vi "ReadDriveEncoder.vi"() -> ()   [LabVIEW 2013]
uses:
  RefnameEnum.ctl
  Sally_Dashboard_2014/DBNameEnum.ctl
  Robot Global Data.vi
panel:
  out "DistanceR (in)":dbl
  out "EncoderR Rate (deg/sec)":dbl
  in  "Reset EncoderR?":bool
  in  "Reset EncoderL?":bool
  out "EncoderL Rate (deg/sec)":dbl
  out "DistanceL (in)":dbl
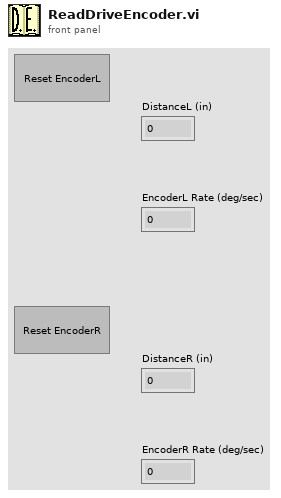
[diagram p1: front panel]
types:
  T1 = typedef "RefnameEnum.ctl" = enum16{"FireLauncher", "Climber", "Shield", "TankDrive", "DriveEncoderL", "DriveEncoderR", "LauncherMotorRPM", "LauncherEncoderAnalog", "LauncherEncoderRPM", "ShooterLS", "DriveAlignLSLeft", "DriveAlignLSRight", "ClimbingLS", "LauncherEncoderAngle", "LauncherMotorAngle", "Gamepad1", "Gamepad2", "Compressor", "ClimbWeightSol3", "ClimbWeightSol4"}
  T2 = typedef "WPI_EncoderDevRef.ctl" = cluster{"DevStatus":errorcluster, "EncoderIndex":T3, "CounterIndex":T4, "DistancePerCount":dbl, "Decoding Type":T5}
  T3 = typedef "FPGA_EncoderIdx.ctl" = enum8{"Enc 0", "Enc 1", "Enc 2", "Enc 3", "Invalid"}
  T4 = typedef "FPGA_CounterCtrSystemIndex.ctl" = enum8{"Ctr 0", "Ctr 1", "Ctr 2", "Ctr 3", "Ctr 4", "Ctr 5", "Ctr 6", "Ctr 7", "Invalid"}
  T5 = typedef "WPI_EncoderType.ctl" = enum16{"1x", "2x", "4x"}
  T6 = typedef "DBNameEnum.ctl" = enum16{"AutoInstructions", "DriveLoopTime", "DriveAlignLSLeft", "DriveAlignLSRight", "Use2DriveAlign", "ClimbLS", "LauncherAngleMatches", "FrameworkVersion", "sLauncherAngle", "LauncherTargetAngle", "sLauncherRPM", "LauncherTargetRPM", "sDriveDistance", "LauncherMotorValue", "PullbackTol", "FireTol", "LauncherRPMTol", "LauncherAngleTol", "InitialWait", "WaitBetweenLaunch", "AnglePresets", "RPMPresets", "UseAngleEncoder", "UseLauncherEncoder", "UseLauncherPID", "QSWaitBeforeFire", "QSWaitBeforeRetract", "AngleForwardValue", "AngleBackwardValue", "UseClusterArray", "BackupAuto", "ReverseDriveIndicate", "HalfSpeedFactor"}
  T7 = typedef "LoopDisable.ctl" = cluster{"Climb.vi":bool, "LauncherAngle.vi":bool, "Launcher.vi":bool, "ArmControl.vi":bool, "WinchMotor.vi":bool, "ReadDriveEncoder.vi":bool}
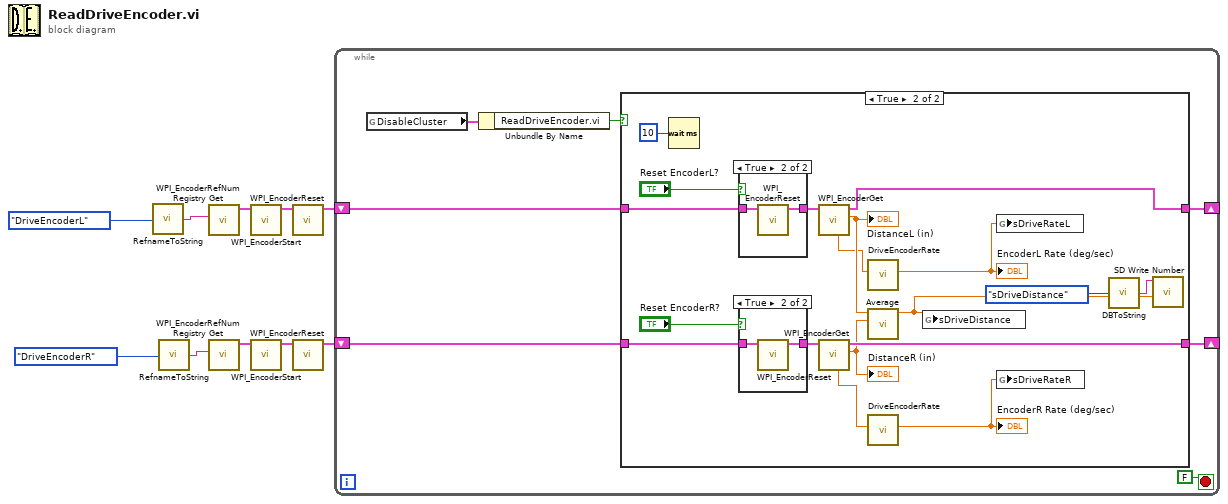
[diagram p0: block diagram]
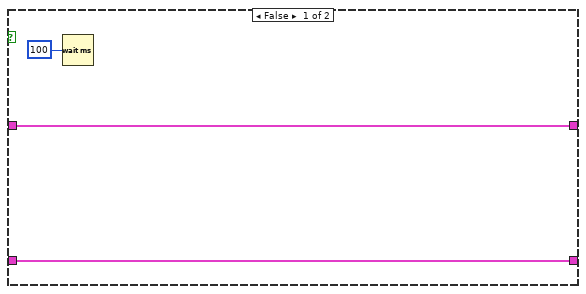
[diagram p2: hidden frame]
diagram:
  n1 = call "RefnameToString.vi"("Enum"=RefnameEnum."DriveEncoderL") -> ("Refname"=w2:string)
  n2 = call "RefnameToString.vi"("Enum"=RefnameEnum."DriveEncoderR") -> ("Refname"=w1:string)
  n3 = call <vilib>:"WPI_EncoderRefNum Registry Get.vi"("refnum name"=w2) -> ("EncoderDevRef"=w10:T2)  [unwired: 9 in, 1 out]
  n4 = call <vilib>:"WPI_EncoderRefNum Registry Get.vi"("refnum name"=w1) -> ("EncoderDevRef"=w7:T2)  [unwired: 9 in, 1 out]
  n5 = call <vilib>:"WPI_EncoderStart.vi"("EncoderDevRef"=w10) -> ("EncoderDevRef"=w9:T2)  [unwired: 1 in, 9 out]
  n6 = call <vilib>:"WPI_EncoderStart.vi"("EncoderDevRef"=w7) -> ("EncoderDevRef"=w6:T2)  [unwired: 1 in, 9 out]
  n7 = call <vilib>:"WPI_EncoderReset.vi"("EncoderDevRef"=w9) -> ("EncoderDevRef"=w8:T2)  [unwired: 1 in, 9 out]
  n8 = call <vilib>:"WPI_EncoderReset.vi"("EncoderDevRef"=w6) -> ("EncoderDevRef"=w5:T2)  [unwired: 1 in, 9 out]
  n9 = while {
    shift-right: [w15] -> _
    shift-left: w8 -> [w16]
    shift-right: [w14] -> _
    shift-left: w5 -> [w13]
    stop <- FALSE stop-if-true
    n10 = global read "Robot Global Data.vi" "DisableCluster"() -> (w12:T7)
    n11 = Unbundle By Name(w12) -> ("ReadDriveEncoder.vi"=w11:bool)
    n12 = case shown="True" w11 {
      tunnel: w16 -> [w20 w37]
      tunnel: [w20 w35] -> w15
      tunnel: [w19 w33] -> w14
      tunnel: w13 -> [w19 w32]
      frame False {
        n13 = Wait (ms)(milliseconds to wait=u32 100) -> ()  [unwired: 1 out]
      }
      frame True {
        n14 = Wait (ms)(milliseconds to wait=u32 10) -> ()  [unwired: 1 out]
        n15 = case shown="True" "Reset EncoderL?" {
          tunnel: w37 -> [w42 w44]
          tunnel: [w42 w43] -> w36
          frame False {
          }
          frame True {
            n16 = call <vilib>:"WPI_EncoderReset.vi"("EncoderDevRef"=w44) -> ("EncoderDevRef"=w43:T2)  [unwired: 9 in, 1 out]
          }
        }
        n17 = case shown="True" "Reset EncoderR?" {
          tunnel: [w39 w41] -> w30
          tunnel: w32 -> [w39 w40]
          frame False {
          }
          frame True {
            n18 = call <vilib>:"WPI_EncoderReset.vi"("EncoderDevRef"=w40) -> ("EncoderDevRef"=w41:T2)  [unwired: 9 in, 1 out]
          }
        }
        n19 = call <vilib>:"WPI_EncoderGet.vi"("EncoderDevRef"=w36) -> ("Distance"=w29:dbl, "EncoderDevRef"=w35:T2, "Rate"=w27:dbl)  [unwired: 5 in, 3 out]
        "DistanceL (in)" <- w29
        n20 = call <vilib>:"WPI_EncoderGet.vi"("EncoderDevRef"=w30) -> ("Distance"=w28:dbl, "EncoderDevRef"=w33:T2, "Rate"=w25:dbl)  [unwired: 5 in, 3 out]
        "DistanceR (in)" <- w28
        n21 = call "DriveEncoderRate.vi"("EncoderRate"=w27) -> ("RateOut"=w26:dbl)  [unwired: 10 in]
        "EncoderL Rate (deg/sec)" <- w26
        n22 = call "Average.vi"("y"=w28, "x"=w29) -> ("x/y"=w21:dbl)  [unwired: 9 in]
        n23 = call "DriveEncoderRate.vi"("EncoderRate"=w25) -> ("RateOut"=w24:dbl)  [unwired: 10 in]
        "EncoderR Rate (deg/sec)" <- w24
        n24 = global write "Robot Global Data.vi" "sDriveDistance"(w21) -> ()
        n25 = global write "Robot Global Data.vi" "sDriveRateL"(w26) -> ()
        n26 = global write "Robot Global Data.vi" "sDriveRateR"(w24) -> ()
        n27 = call "DBToString.vi"("Enum"=DBNameEnum."sDriveDistance") -> ("Refname"=w22:string)
        n28 = call <vilib>:"SD Write Number.vi"("Numeric"=w21, "Name"=w22) -> ()  [unwired: 8 in, 2 out]
      }
    }
  }
